vi "Send Set Expected Heartbeat Entry.vi"(7 "Message Priority (Normal)":T2=enum."Normal", 8 "error in (no error)":errorcluster, 9 "Entry":T1 {"Last Beat" format="%<%x %.3X>T"; "Timeout" format="%d ms"; "Period" format="%d ms"}, 10 "Node-ID":u8, 11 "Message Enqueuer":refnum<class "Message Enqueuer.lvclass">) -> (0 "error out":errorcluster, 3 "Message Enqueuer out":refnum<class "Message Enqueuer.lvclass">)   [LabVIEW 2024, in "Network Management UI.lvlib" / "Set Expected Heartbeat Entry Msg.lvclass"]
doc: "This VI sends the message to an actor."
uses:
  Set Expected Heartbeat Entry Msg.lvclass
  <vilib>/ActorFramework/Message Enqueuer/Message Enqueuer.lvclass
  <vilib>/ActorFramework/Message Enqueuer/Message Priority.ctl
  C:/Program Files/National Instruments/LabVIEW 2025/vi.lib/ActorFramework/Message/Message.lvclass
  Set Expected Heartbeat Entry Msg.lvclass/Set Expected Heartbeat Entry Msg.ctl
  <vilib>/ActorFramework/Message Enqueuer/Message Enqueuer.lvclass/Message Enqueuer.ctl
  <vilib>/Utility/LVClass/Get LV Class Name.vi
  <vilib>/ActorFramework/tracing/Trace Generation/Generate Trace for Message.vi
  <vilib>/ActorFramework/Message Priority Queue/Priority Enqueue.vi
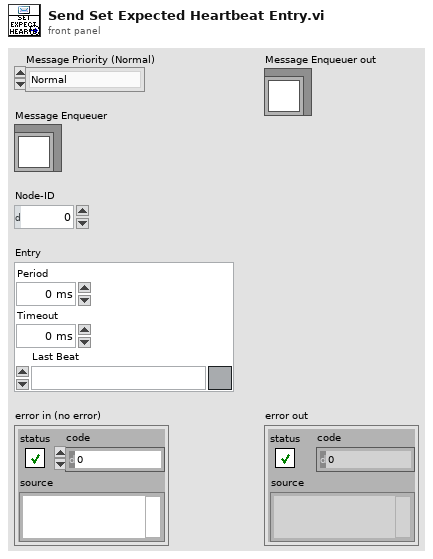
[diagram p1: front panel]
types:
  T1 = cluster{"Period":u16, "Timeout":u16, "Last Beat":timestamp}
  T2 = typedef "Actor Framework.lvlib/Message Enqueuer.lvclass/Message Priority.ctl" = enum16{"Low", "Normal", "High"}
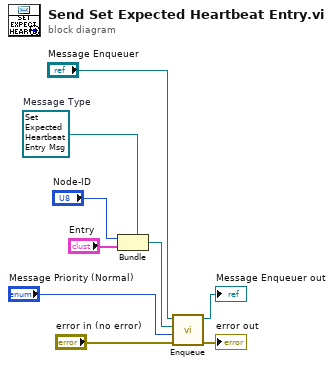
[diagram p0: block diagram]
diagram:
  w3 = refnum<class "Set Expected Heartbeat Entry Msg.lvclass"> refnum  # Message Type
  n1 = Bundle(cluster=w3, "Node-ID", "Entry") -> (w4:refnum<class "Set Expected Heartbeat Entry Msg.lvclass">)
  n2 = call <vilib>:"Enqueue.vi"("error in (no error)"="error in (no error)", "Message Priority (Normal)"="Message Priority (Normal)", "Message"=w4, "Message Enqueuer in"="Message Enqueuer") -> ("error out"=→"error out":errorcluster, "Message Enqueuer out"=→"Message Enqueuer out":refnum<class "Message Enqueuer.lvclass">)  [unwired: 6 in]
